vi "MCL Level Z.vi"(10 "handle":i32, 11 "position":dbl) -> (3 "function return":i32)   [LabVIEW 2017, in "Madlib.lvlib"]
doc: "MADLIB_API int MCL_LevelZ(double position, int handle);"
uses:
  Madlib.lvlib
  Madlib.dll
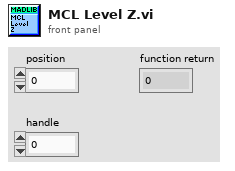
[diagram p1: front panel]
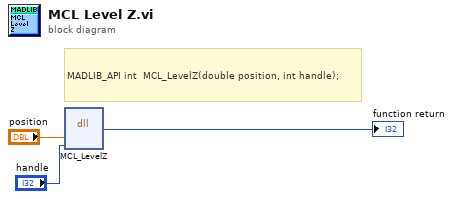
[diagram p0: block diagram]
diagram:
  # "MADLIB_API\tint\t\tMCL_LevelZ(double position, int handle);"
  n1 = dll-call lib="C:/Users/francesco/dev/pump-probe/Piezo/lvlib/Madlib.*" fn="MCL_LevelZ"("position"="position", "handle"="handle") -> (→"function return":i32)  [unwired: 5 in, 2 out]
